vi "Get_VI_Path.vi"() -> (0 "path":path)   [LabVIEW 2018]
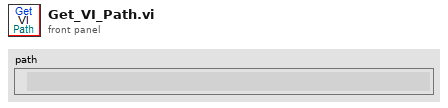
[diagram p1: front panel]
types:
  T1 = enum32{"invalid app kind", "Development System", "Run Time System", "Student Edition", "Embedded LabVIEW", "Evaluation", "Custom"}
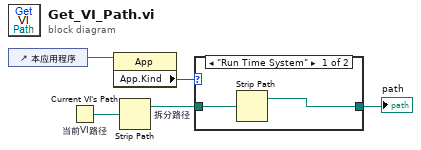
[diagram p0: block diagram]
diagram:
  n1 = control-ref of="本应用程序"() -> (w5:refnum<vi>)
  n2 = Current VI's Path "当前VI路径"() -> (path=w3:path)
  n3 = property class="App"(reference=w5) -> ("App.Kind"=w4:T1)  [unwired: 1 in, 2 out]
  n4 = Strip Path "拆分路径"(path=w3) -> (stripped path=w2:path)  [unwired: 1 out]
  n5 = case shown="\"Run Time System\"" w4 {
    tunnel: w2 -> [w7 w8]
    tunnel: [w6 w8] -> w1
    frame "Run Time System" {
      n6 = Strip Path(path=w7) -> (stripped path=w6:path)  [unwired: 1 out]
    }
    frame "Development System", Default {
    }
  }
  "path" <- w1
